vi "Derivative.vi"(8 "error in (no error)":errorcluster, 11 "PID in":refnum<class "PID.lvclass">) -> (0 "error out":errorcluster, 3 "PID out":refnum<class "PID.lvclass">)   [LabVIEW 2024, in "PID.lvlib" / "PID.lvclass"]
uses:
  PID.lvclass
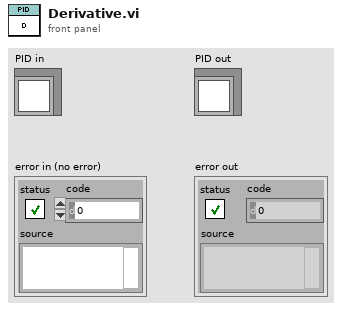
[diagram p1: front panel]
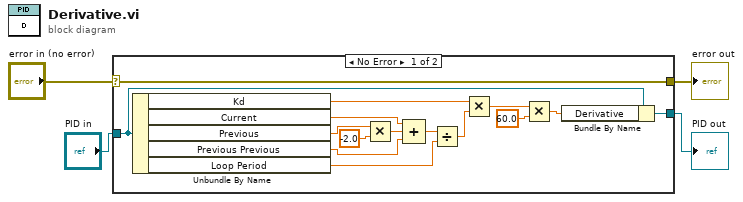
[diagram p0: block diagram]
diagram:
  n1 = case shown="No Error" "error in (no error)" {
    selector: "error in (no error)" -> [w19 w21]
    tunnel: [w19 w21] -> w3
    tunnel: [w5 w20] -> w1
    tunnel: "PID in" -> [w7 w20]
    frame No Error {
      n2 = Unbundle By Name(w7) -> ("Kd"=w11:dbl, "Current"=w16:dbl, "Previous"=w18:dbl, "Previous Previous"=w14:dbl, "Loop Period"=w12:dbl)
      n3 = Multiply(x=w18, y=-2.0) -> (x*y=w15:dbl)
      n4 = Compound Arithmetic op=ADD(w16, w15, w14) -> (w13:dbl)
      n5 = Divide(x=w13, y=w12) -> (x/y=w10:dbl)
      n6 = Multiply(x=w11, y=w10) -> (x*y=w9:dbl)
      n7 = Multiply(x=w9, y=60.0) -> (x*y=w6:dbl)
      n8 = Bundle By Name(cluster=w7, "Derivative"=w6) -> (w5:refnum<class "PID.lvclass">)
    }
    frame Error {
    }
  }
  "error out" <- w3
  "PID out" <- w1
